vi "Check if Package Exists in SystemLink Repository.vi"(0 "SystemLink repo in":T1, 7 "package name":string, 9 "pacakge version":string, 11 "error in (no error)":errorcluster) -> (4 "SystemLink repo out":T1, 8 "exists?":bool, 15 "error out":errorcluster)   [LabVIEW 2017, in "SystemLink_Repo_API.lvlib"]
doc: "Check if the package and version exists in the SystemLink repository."
uses:
  SystemLink_Repo_API.lvlib
  _support/systemlink repo.ctl
  <vilib>/httpClient/ClientHandle.ctl
  <vilib>/httpClient/LabVIEWHTTPClient.lvlib
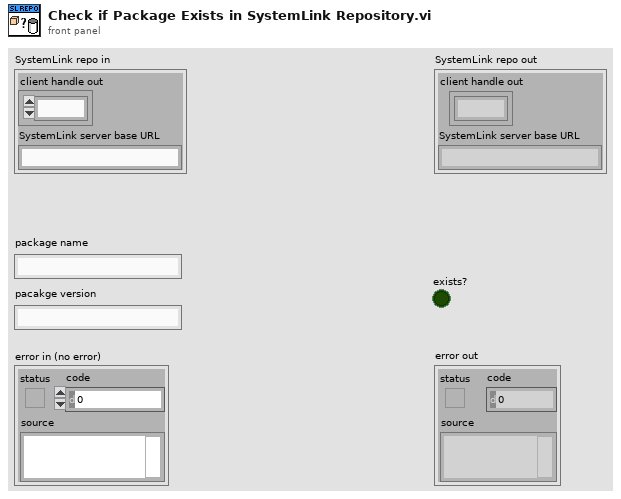
[diagram p1: front panel]
types:
  T1 = typedef "SystemLink_Repo_API.lvlib/systemlink repo.ctl" = cluster{"client handle out":T2, "SystemLink server base URL":string}
  T2 = typedef "LabVIEWHTTPClient.lvlib/ClientHandle.ctl" = refnum<k1>
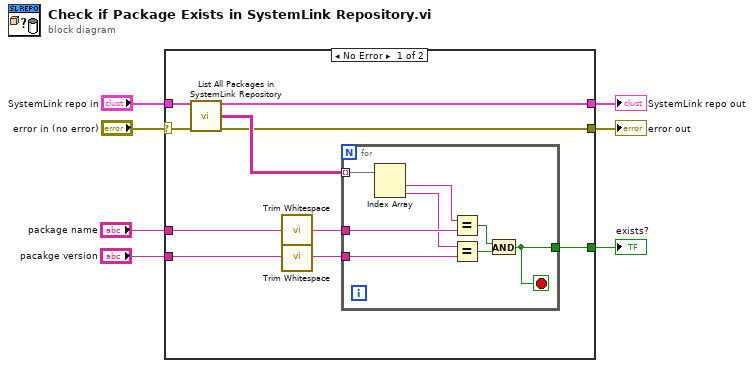
[diagram p0: block diagram]
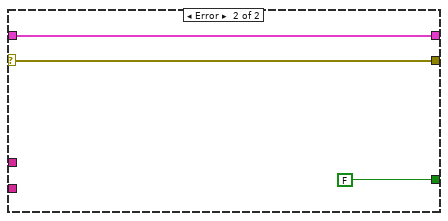
[diagram p2: hidden frame]
diagram:
  n1 = case shown="No Error" "error in (no error)" {
    selector: "error in (no error)" -> [w9 w28]
    tunnel: "SystemLink repo in" -> [w12 w27]
    tunnel: [w8 w28] -> w5
    tunnel: [w11 w27] -> w4
    tunnel: [w13 FALSE ("timed out?")] -> w3
    tunnel: "package name" -> [w17 _]
    tunnel: "pacakge version" -> [w16 _]
    frame No Error {
      n2 = call "List All Packages in SystemLink Repository.vi"("SystemLink repo in"=w12, "error in (no error)"=w9) -> ("SystemLink repo out"=w11:T1, "packages"=w10:string[][], "error out"=w8:errorcluster)  [unwired: 11 in]
      n3 = call <vilib>:"Trim Whitespace.vi"("string"=w17) -> ("trimmed string"=w15:string)  [unwired: 1 in]
      n4 = call <vilib>:"Trim Whitespace.vi"("string"=w16) -> ("trimmed string"=w14:string)  [unwired: 1 in]
      n5 = for {
        tunnel: w10 -> [w25] mode=indexing
        tunnel: w15 -> [w23]
        tunnel: w14 -> [w21]
        tunnel: [w18] -> w13
        stop <- w18 stop-if-true
        n6 = Index Array(array=w25) -> (element #1=w24:string, element #2=w22:string)  [unwired: 2 in]
        n7 = Equal?(x=w24, y=w23) -> (x = y?=w20:bool)
        n8 = Equal?(x=w22, y=w21) -> (x = y?=w19:bool)
        n9 = And(x=w20, y=w19) -> (x .and. y?=w18:bool)
      }
    }
    frame Error {
    }
  }
  "error out" <- w5
  "SystemLink repo out" <- w4
  "exists?" <- w3
